vi "MenuDo.vi"(4 "ModeCol Index":i32=2, 6 "Cell Position":T2, 8 "error in (no error)":errorcluster, 9 "SetList Refs":T1, 10 "ItemTag":string, 11 "MenuCol in":refnum<class "MenuCol.lvclass">) -> (0 "error out":errorcluster, 1 "Table CtlRef Out":refnum<vi>, 2 "Col Array Ref out":refnum<vi>, 3 "MenuCol out":refnum<class "MenuCol.lvclass">, 5 "Update HWI?":bool)   [LabVIEW 2013, in "MenuCol.lvclass"]
doc: "Perform selected shortcut (right-click) menu actions for all columns in general.\nThis VI is read-only w.r.t column data."
uses:
  MenuCol.lvclass
  Column/Column.lvclass
  <vilib>/Utility/miscctls.llb/LVRowAndColumnTypeDef.ctl
  TypeDefs/TableArray.ctl
  TypeDefs/TableHistory.ctl
  VariableManagerCodes/VariableManager/VariableManager.lvclass
  TypeDefs/SetListRefs.ctl
  DeviceVIs/Device/Device.lvclass
  Utils/InsertMenu/InsertFunctionMenu.lvclass
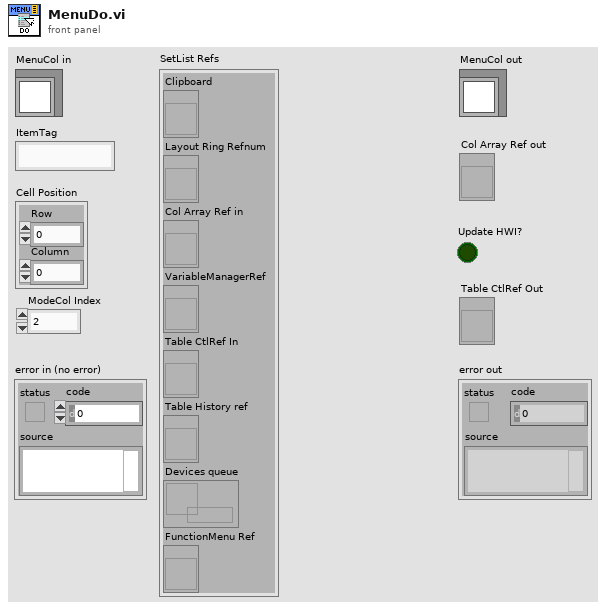
[diagram p1: front panel]
types:
  T1 = typedef "SetListRefs.ctl" = cluster{"Clipboard":refnum<vi>, "Layout Ring Refnum":refnum<vi>, "Col Array Ref in":refnum<vi>, "VariableManagerRef":refnum<vi>, "Table CtlRef In":refnum<vi>, "Table History ref":refnum<vi>, "Devices queue":refnum<queue>, "FunctionMenu Ref":refnum<vi>}
  T2 = typedef "LVRowAndColumnTypeDef.ctl" = cluster{"Row":i32, "Column":i32}
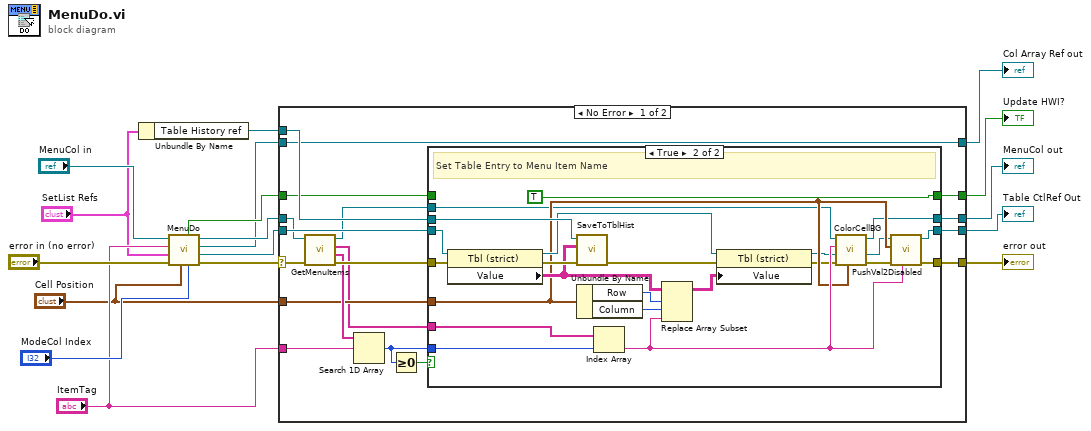
[diagram p0: block diagram]
diagram:
  n1 = Unbundle By Name("SetList Refs") -> ("Table History ref"=w1:refnum<vi>)
  n2 = call-parent "MenuDo.vi"("ModeCol Index"="ModeCol Index", "Cell Position"="Cell Position", "error in (no error)"="error in (no error)", "SetList Refs"="SetList Refs", "ItemTag"="ItemTag", "Column in"="MenuCol in") -> ("error out"=w10:errorcluster, "Table CtlRef Out"=w8:refnum<vi>, "Col Array Ref out"=w4:refnum<vi>, "Column out"=w12:refnum<class "MenuCol.lvclass">, "Update HWI?"=w14:bool)  [unwired: 1 in]
  n3 = case shown="No Error" w10 {
    selector: w10 -> [w35 w67]
    tunnel: [w26 w67] -> w6
    tunnel: "ItemTag" -> [w34 _]
    tunnel: w1 -> [w31 _]
    tunnel: "Cell Position" -> [w30 _]
    tunnel: [w27 w65] -> w7
    tunnel: [w18 w66] -> w5
    tunnel: w8 -> [w24 w65]
    tunnel: w12 -> [w23 w66]
    tunnel: w4 -> [w22 w64]
    tunnel: [w22 w64] -> w3
    tunnel: w14 -> [w21 w63]
    tunnel: [w20 w63] -> w13
    frame No Error {
      n4 = call-dynamic "GetMenuItems.vi"("error in (no error)"=w35, "MenuCol in"=w23) -> ("error out"=w33:errorcluster, "MenuTags"=w32:string[], "MenuLabels"=w29:string[], "MenuCol out"=w19:refnum<class "MenuCol.lvclass">)  [unwired: 6 in]
      n5 = Search 1D Array(1D array=w32, element=w34) -> (index of element=w28:i32)  [unwired: 1 in]
      n6 = Greater Or Equal To 0?(x=w28) -> (x >= 0?=w25:bool)
      n7 = case shown="True" w25 {
        tunnel: w33 -> [w39 w62]
        tunnel: w31 -> [_ w60]
        tunnel: w30 -> [_ w46]
        tunnel: w29 -> [_ w56]
        tunnel: w28 -> [_ w55]
        tunnel: [w38 w49] -> w27
        tunnel: [w39 w48] -> w26
        tunnel: w24 -> [w38 w51]
        tunnel: w21 -> [w37 _]
        tunnel: [w37 TRUE ("Update HWI?")] -> w20
        tunnel: w19 -> [w36 w41]
        tunnel: [w36 w40] -> w18
        frame False {
          # "Don't do anything for unexpected entries"
        }
        frame True {
          # "Set Table Entry to Menu Item Name"
          n8 = property class="Tbl (strict)"(reference=w51, error in=w62) -> (reference out=w54:refnum<vi>, error out=w61:errorcluster, "Value"=w58:string[][])
          n9 = call "SaveToTblHist.vi"("error in (no error)"=w61, "OldTable (reset)"=w58, "Table History ref"=w60) -> ("error out"=w53:errorcluster)  [unwired: 8 in]
          n10 = Unbundle By Name(w46) -> ("Row"=w59:i32, "Column"=w57:i32)
          n11 = Index Array(array=w56, index=w55) -> (element=w47:string)
          n12 = Replace Array Subset(array=w58, new element=w47, index (row)=w59, index (col)=w57) -> (w52:string[][])
          n13 = property class="Tbl (strict)"(reference=w54, error in=w53, "Value"=w52) -> (reference out=w42:refnum<vi>, error out=w45:errorcluster)
          n14 = call-dynamic "ColorCellBG.vi"("Cell Position"=w46, "error in (no error)"=w45, "Table CtlRef In"=w42, "Value"=w47, "MenuCol in"=w41) -> ("error out"=w44:errorcluster, "Table CtlRef Out"=w43:refnum<vi>, "MenuCol out"=w40:refnum<class "MenuCol.lvclass">)  [unwired: 4 in]
          n15 = call "PushVal2Disabled.vi"("Value"=w47, "error in (no error)"=w44, "Cell Position"=w46, "Table CtlRef In"=w43) -> ("error out"=w48:errorcluster, "Table CtlRef Out"=w49:refnum<vi>)  [unwired: 5 in, 1 out]
        }
      }
    }
    frame Error {
    }
  }
  "error out" <- w6
  "MenuCol out" <- w5
  "Table CtlRef Out" <- w7
  "Col Array Ref out" <- w3
  "Update HWI?" <- w13
